vi "Create Process.vi"(5 "use stderr (F)":bool, 7 "hide window (T)":bool=TRUE, 8 "error in":errorcluster, 9 "path to lv_proc.dll":path, 10 "command":string, 11 "working folder":string) -> (0 "error out":errorcluster, 3 "pipe handle":T1)   [LabVIEW 2013]
doc: "Calls lv_proc.dll function to create a new process and return pipe handle. Even if the process instance has returned exit code the handle must be closed by proc_cleanup.vi. Process is started by 'command' in 'working folder', and window is hidden if selected. Standard error can be used."
uses:
  Pipe Handle.ctl
  <vilib>/Utility/error.llb/Error Cluster From Error Code.vi
  <vilib>/ErrorRing/Error Ring.xnode
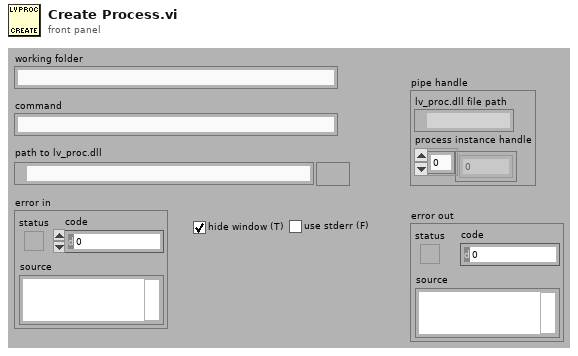
[diagram p1: front panel]
types:
  T1 = typedef "Pipe Handle.ctl" = cluster{"lv_proc.dll file path":path, "process instance handle":u32[]}
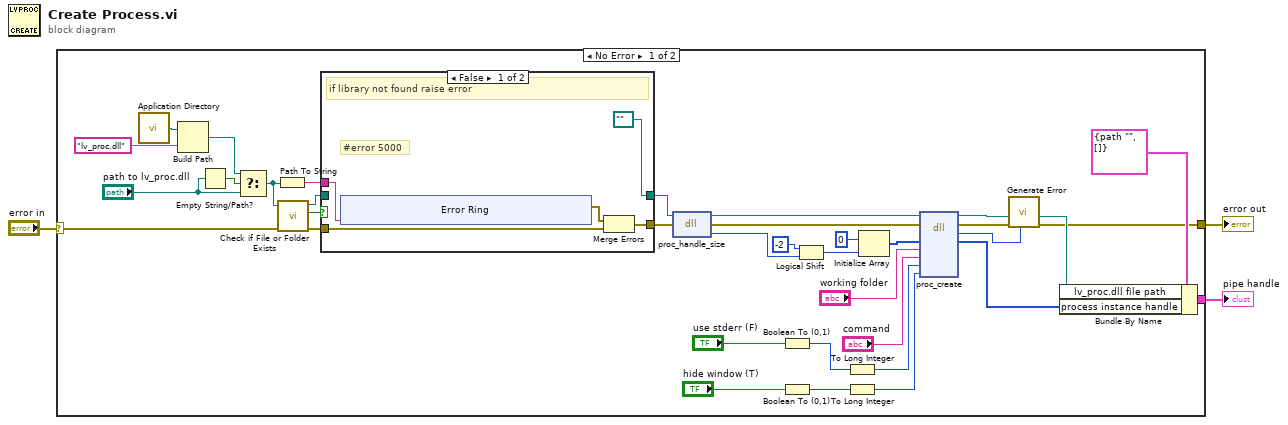
[diagram p0: block diagram]
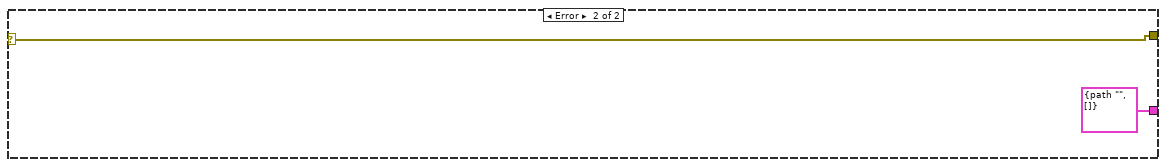
[diagram p3: hidden frame]
diagram:
  n1 = case shown="No Error" "error in" {
    selector: "error in" -> [w28 w55]
    tunnel: [w4 w55] -> w2
    tunnel: [w10 T1 {"lv_proc.dll file path"=path "", "process instance handle"=[]} ("pipe handle out")] -> w1
    frame No Error {
      n2 = call <vilib>:"Application Directory.vi"() -> ("Application Directory"=w34:path)
      n3 = Build Path(base path=w34, name or relative path="lv_proc.dll") -> (appended path=w35:path)
      n4 = Empty String/Path?(string/path="path to lv_proc.dll") -> (empty?=w32:bool)
      n5 = Select(t=w35, s=w32, f="path to lv_proc.dll") -> (s? t:f=w29:path)
      n6 = Path To String(path=w29) -> (string=w30:string)
      n7 = call <vilib>:"Check if File or Folder Exists.vi"("error in (no error)"=w28, "path"=w29) -> ("error out"=w26:errorcluster, "file or folder exists?"=w27:bool, "dup path"=w12:path)  [unwired: 7 in]
      n8 = case shown="False" w27 {
        tunnel: w30 -> [w44 _]
        tunnel: w26 -> [w42 w53]
        tunnel: [w41 w53] -> w17
        tunnel: [path "" ("dup path") w52] -> w13
        tunnel: w12 -> [_ w52]
        frame False {
          # "#error 5000"
          # "if library not found raise error"
          n9 = xnode "Error Ring"("parameter 0"=w44) -> ("error out"=w43:errorcluster)
          n10 = Merge Errors(w43, w42) -> (w41:errorcluster)
        }
        frame True {
        }
      }
      n11 = dll-call lib="lv_proc.dll" fn="proc_handle_size"(path in=w13, error in=w17) -> (path out=w14:path, error out=w15:errorcluster, "size [B]"=w21:i32)  [unwired: 1 in]
      n12 = Boolean To (0,1)(Boolean="use stderr (F)") -> (0, 1=w23:i16)
      n13 = Boolean To (0,1)(Boolean="hide window (T)") -> (0, 1=w25:i16)
      n14 = Logical Shift(y=-2 ("x"), x=w21) -> (x << y=w19:i32)
      n15 = To Long Integer(number=w23) -> (32bit integer=w22:i32)
      n16 = To Long Integer(number=w25) -> (32bit integer=w24:i32)
      n17 = Initialize Array(u32 0 ("element"), w19) -> (w16:u32[])
      n18 = dll-call lib="lv_proc.dll" fn="proc_create"(path in=w14, error in=w15, "proc"=w16, "folder"="working folder", "command"="command", "use_stderr"=w22, "hide_window"=w24) -> (path out=w7:path, error out=w6:errorcluster, "error"=w11:i32, "proc"=w8:u32[])  [unwired: 5 in]
      n19 = call "Generate Error.vi"("error code in"=w11, "error in"=w6, "lv_proc.dll path in"=w7) -> ("error out"=w4:errorcluster, "lv_proc.dll path out"=w5:path)  [unwired: 6 in]
      n20 = Bundle By Name(cluster=T1 {"lv_proc.dll file path"=path "", "process instance handle"=[]} ("pipe"), "lv_proc.dll file path"=w5, "process instance handle"=w8) -> (w10:T1)
    }
    frame Error {
    }
  }
  "error out" <- w2
  "pipe handle" <- w1
